vi "Tokenizer speed test.vi"() -> ()   [LabVIEW 2019]
uses:
  PathTokenizer/PathTokenizer.lvclass
  PathTokenizer/PathTokenizer.lvclass/PathTokenizer.ctl
panel:
  out "Tokens":string[](array[string])
  out "x/y":dbl
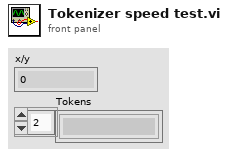
[diagram p1: front panel]
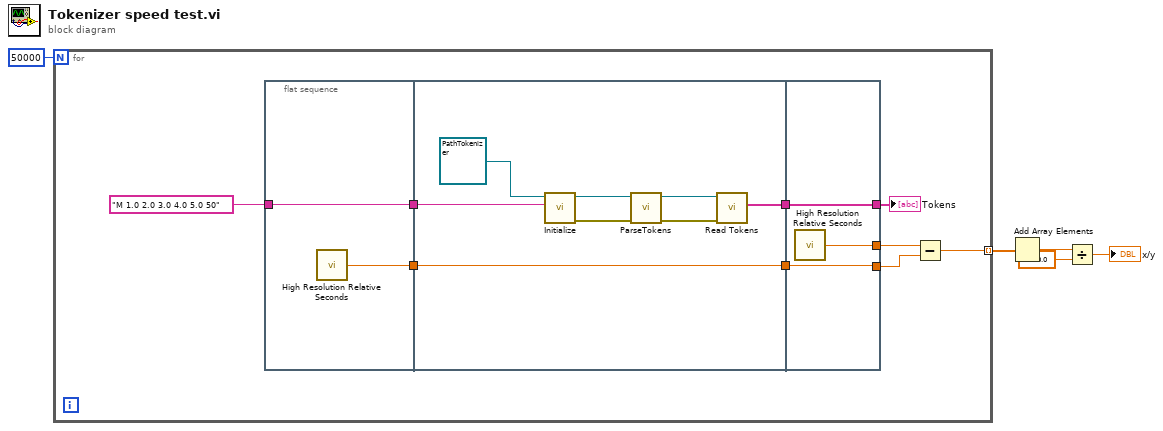
[diagram p0: block diagram]
diagram:
  n1 = for {
    N: 50000 -> [_]
    tunnel: [w7] -> w5 mode=indexing
    n2 = flat-sequence {
      tunnel: [w16] -> w14
      tunnel: "M 1.0 2.0 3.0 4.0 5.0 50" ("Path Command Text") -> [w16]
      tunnel: [w15] -> w13
      tunnel: w14 -> [w19]
      tunnel: [w18] -> w12
      tunnel: [w17] -> w11
      tunnel: w13 -> [w17]
      tunnel: [w27] -> w6
      tunnel: w12 -> [w27]
      tunnel: w11 -> [w25]
      tunnel: [w26] -> w9
      tunnel: [w25] -> w8
      frame #0 {
        n3 = call <vilib>:"High Resolution Relative Seconds.vi"() -> ("relative seconds"=w15:dbl)
      }
      frame #1 {
        n4 = call "Initialize.vi"("Path Command Text"=w19, "PathTokenizer in"=refnum<class "PathTokenizer.lvclass"> refnum) -> ("error out"=w23:errorcluster, "PathTokenizer out"=w24:refnum<class "PathTokenizer.lvclass">)  [unwired: 8 in]
        n5 = call "ParseTokens.vi"("error in (no error)"=w23, "PathTokenizer in"=w24) -> ("error out"=w21:errorcluster, "PathTokenizer out"=w22:refnum<class "PathTokenizer.lvclass">)  [unwired: 8 in]
        n6 = call "Read Tokens.vi"("error in (no error)"=w21, "PathTokenizer in"=w22) -> ("Tokens"=w18:string[])  [unwired: 7 in, 2 out]
      }
      frame #2 {
        n7 = call <vilib>:"High Resolution Relative Seconds.vi"() -> ("relative seconds"=w26:dbl)
      }
    }
    n8 = Subtract(x=w9, y=w8) -> (x-y=w7:dbl)
    "Tokens" <- w6
  }
  n9 = Add Array Elements(numeric array=w5) -> (sum=w4:dbl)
  n10 = Divide(x=w4, y=50000.0) -> (x/y=→"x/y":dbl)
